vi "Test Depth.vi"() -> ()   [LabVIEW 2015]
uses:
  Controls/Led Control.ctl
  <vilib>/Analysis/baseanly.llb/Mean (DBL).vi
  <vilib>/myRIO/Common/Instrument Driver Framework/myRIO v1.0/UART/vis/myRIO v1.0 Close UART.vi
  <vilib>/myRIO/Common/Instrument Driver Framework/Utilities/vis/FPGA Ref Manager.vi
  <vilib>/myRIO/Common/Instrument Driver Framework/myRIO v1.0/myRIO v1.0 Reset FPGA.vi
  <vilib>/myRIO/Common/Instrument Driver Framework/myRIO v1.0/IRQ/vis/myRIO v1.0 IRQ Info FGV.vi
  <vilib>/myRIO/Common/Instrument Driver Framework/myRIO v1.0/IRQ/vis/myRIO v1.0 Timer IRQ Info FGV.vi
  <vilib>/myRIO/Common/Instrument Driver Framework/myRIO v1.0/IRQ/vis/myRIO v1.0 ISR Agent.vi
  <vilib>/myRIO/Instrument Drivers/Utilities/Utilities.lvlib
  <vilib>/Analysis/NI_AALBase.lvlib
panel:
  out "mean":dbl format="%0.2f"
  out "period":u32
  out "error out":errorcluster
  in  "Led Option":T1=enum."LED_RED"
  in  "tilt degree":i32=12
  in  "Depth Format":T2(ring)=enum."FREENECT_DEPTH_10BIT"
  in  "stop":bool
  out "Depth":T3(plugin-control)
  in  "Size":enum16{"Low (320x240)", "Tiny (160x120)"}(ring)
  # "Low--->8,5 ms\nTiny--->2,5 ms"
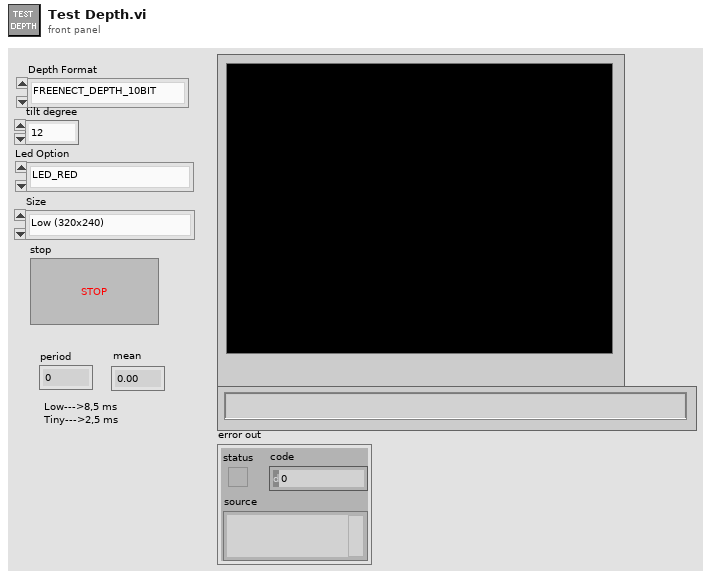
[diagram p1: front panel]
types:
  T1 = typedef "Led Control.ctl" = enum32{"LED_OFF", "LED_GREEN", "LED_RED", "LED_YELLOW", "LED_BLINK_GREEN", "LED_BLINK_GREEN2", "LED_BLINK_RED_YELLOW"}
  T2 = enum32{"FREENECT_DEPTH_11BIT", "FREENECT_DEPTH_10BIT", "FREENECT_DEPTH_11BIT_PACKED", "FREENECT_DEPTH_10BIT_PACKED", "FREENECT_DEPTH_REGISTERED", "FREENECT_DEPTH_MM"}
  T3 = typedef "IMAQ Image.ctl" = refnum<image>
  T4 = typedef "Image Type" = u32
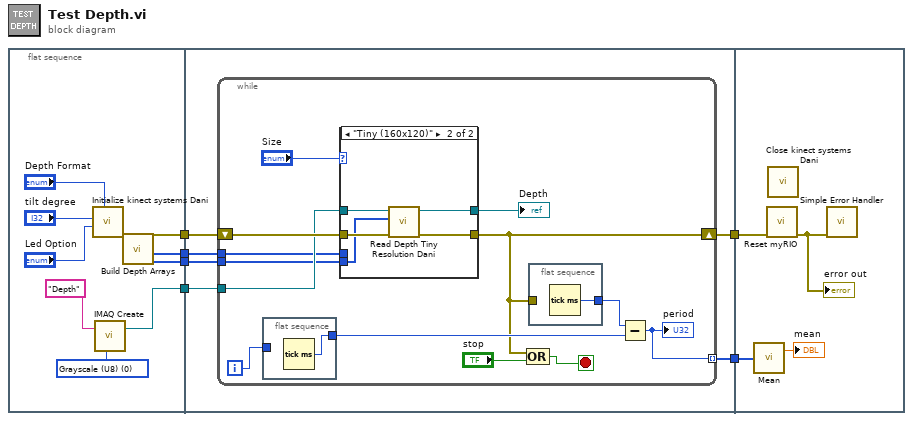
[diagram p0: block diagram]
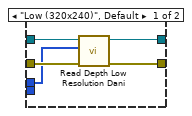
[diagram p2: hidden frame]
diagram:
  n1 = flat-sequence {
    tunnel: [w15] -> w6
    tunnel: [w14] -> w4
    tunnel: [w8] -> w3
    tunnel: [w7] -> w2
    tunnel: w6 -> [w21]
    tunnel: [w20] -> w5
    tunnel: w4 -> [w19]
    tunnel: w3 -> [w18]
    tunnel: w2 -> [w17]
    tunnel: [w16] -> w1
    tunnel: w5 -> [w50]
    tunnel: w1 -> [w48]
    frame #0 {
      w9 = T4 0 items=["Grayscale (U8)", "Grayscale (I16)", "Grayscale (SGL)", "Complex (CSG)", "RGB (U32)", "HSL (U32)", "RGB (U64)", "Grayscale (U16)"] ("Image Type")
      n2 = call "Initialize kinect systems Dani.vi"("Depth Format"="Depth Format", "Led Option"="Led Option", "tilt degree"="tilt degree") -> ("error out"=w15:errorcluster)  [unwired: 8 in]
      n3 = call "IMAQ Create"("Image Name"="Depth", "Image Type"=w9) -> ("New Image"=w14:T3)  [unwired: 3 in, 1 out]
      n4 = call "Build Depth Arrays.vi"() -> ("Array Tiny"=w7:u16[], "Array Low"=w8:u16[])  [unwired: 10 in]
    }
    frame #1 {
      n5 = while {
        shift-right: [w23] -> w20
        shift-left: w21 -> [w32]
        tunnel: w19 -> [w29]
        tunnel: w18 -> [w28]
        tunnel: w17 -> [w27]
        tunnel: [w22] -> w16 mode=indexing
        i -> [w26]
        stop <- w30 stop-if-true
        n6 = flat-sequence {
          tunnel: w26 -> [_]
          tunnel: [w36] -> w24
          frame #0 {
            n7 = Tick Count (ms)() -> (millisecond timer value=w36:u32)
          }
        }
        n8 = case shown="\"Tiny (160x120)\"" "Size" {
          tunnel: [w41 w42] -> w33
          tunnel: [w40 w45] -> w23
          tunnel: w32 -> [w39 w46]
          tunnel: w29 -> [w38 w44]
          tunnel: w28 -> [w37 _]
          tunnel: w27 -> [_ w43]
          frame "Low (320x240)", Default {
            n9 = call "Read Depth Low Resolution Dani.vi"("error in (no error)"=w39, "depth"=w37, "Image In"=w38) -> ("error out"=w40:errorcluster, "Image Out"=w41:T3)  [unwired: 7 in]
          }
          frame "Tiny (160x120)" {
            n10 = call "Read Depth Tiny Resolution Dani.vi"("error in (no error)"=w46, "depth"=w43, "Image In"=w44) -> ("error out"=w45:errorcluster, "Image Out"=w42:T3)  [unwired: 7 in]
          }
        }
        "Depth" <- w33
        n11 = Compound Arithmetic op=OR(w23, "stop") -> (w30:bool)
        n12 = flat-sequence {
          tunnel: [w35] -> w25
          tunnel: w23 -> [_]
          frame #0 {
            n13 = Tick Count (ms)() -> (millisecond timer value=w35:u32)
          }
        }
        n14 = Subtract(x=w25, y=w24) -> (x-y=w22:u32)
        "period" <- w22
      }
    }
    frame #2 {
      n15 = call-poly <vilib>:"Mean.vi"("X"=w48) -> ("mean"=→"mean":dbl)  [unwired: 1 out]
      n16 = call <vilib>:"Reset myRIO.vi"("error in (no error)"=w50) -> ("error out"=w49:errorcluster)  [unwired: 10 in]
      "error out" <- w49
      n17 = call "Close kinect systems Dani.vi"() -> ()  [unwired: 11 in, 1 out]
      n18 = call <vilib>:"Simple Error Handler.vi"("error in (no error)"=w49) -> ()  [unwired: 4 in, 5 out]
    }
  }
